vi "pass_2d_to_DLL.vi"() -> ()   [LabVIEW 2015]
panel:
  in  "sir_in":i32[][](array[numeric])
  in  "Unload":bool
  in  "File Path":path=path "C:/Program Files/National Instruments/LabVIEW 2009/examples/dll/hostname/hostname.dll"
  in  "error in":errorcluster
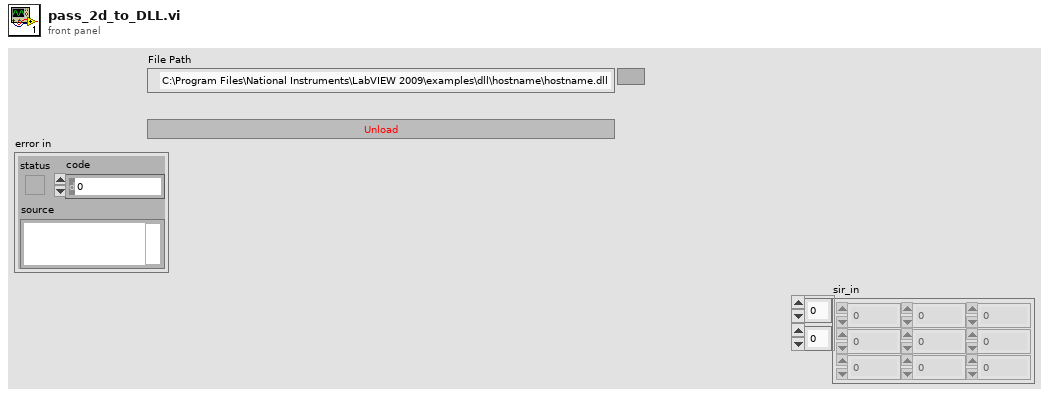
[diagram p1: front panel]
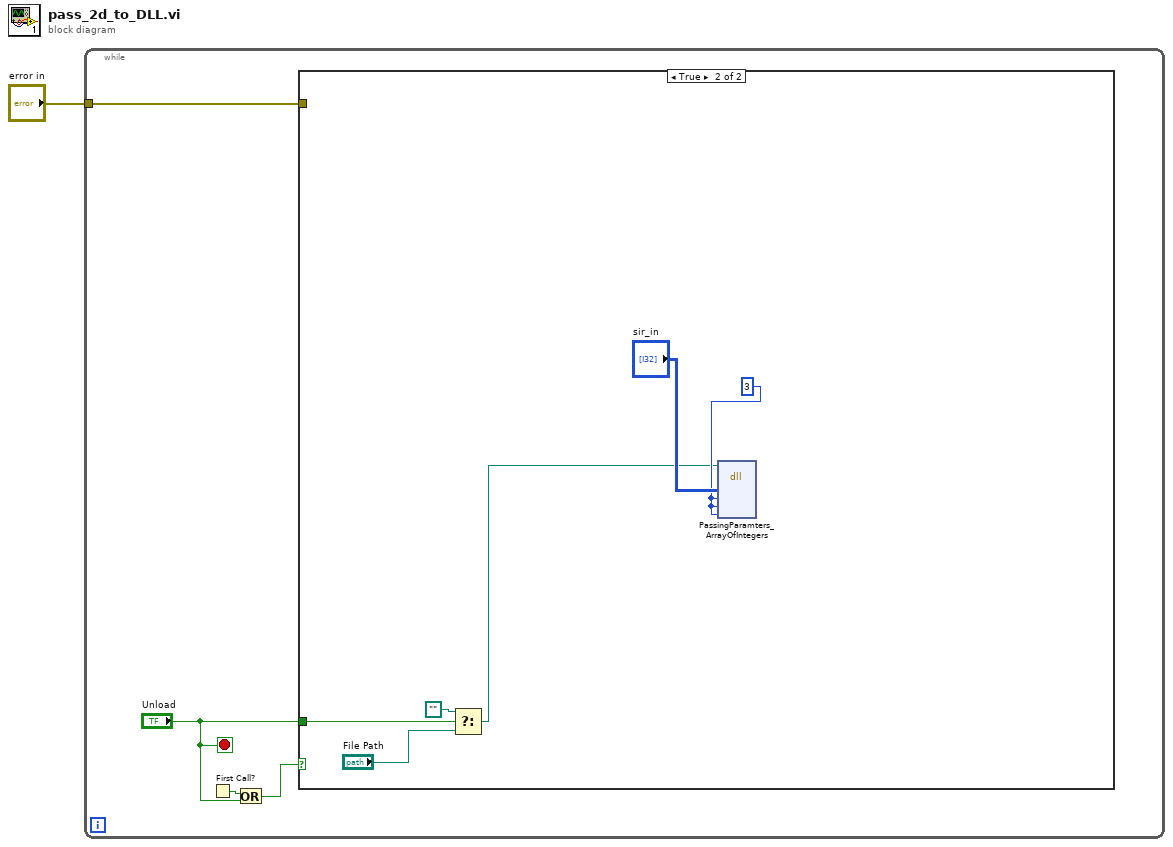
[diagram p0: block diagram]
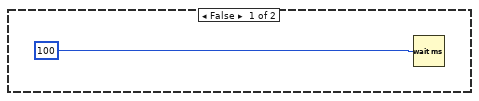
[diagram p2: hidden frame]
diagram:
  n1 = while {
    tunnel: "error in" -> [w2]
    stop <- "Unload" stop-if-true
    n2 = First Call?() -> (First Call?: T/F=w5:bool)
    n3 = Or(x=w5, y="Unload") -> (x .or. y?=w4:bool)
    n4 = case shown="True" w4 {
      tunnel: "Unload" -> [_ w12]
      tunnel: w2 -> [_ _]
      frame False {
        n5 = Wait (ms)(milliseconds to wait=u32 100) -> ()  [unwired: 1 out]
      }
      frame True {
        w8 = 3 ("length")
        n6 = Select(t=path "", s=w12, f="File Path") -> (s? t:f=w7:path)
        n7 = dll-call lib="D:/PROIECT DRONA/BmpWork/pass_array_to_dll/bin/Debug/pass_array_to_dll.dll" fn="PassingParamters_ArrayOfIntegers"(path in=w7, "sir"="sir_in", "length"=w8, "height"=w8, "size"=w8) -> ()  [unwired: 7 in, 2 out]
      }
    }
  }
